vi "SetTextplain.vi"(8 "error in (no error)":errorcluster, 10 "text/plain":string, 11 "object in":refnum<class "execute_result Message.lvclass">) -> (0 "error out":errorcluster, 3 "object out":refnum<class "execute_result Message.lvclass">)   [LabVIEW 2018]
uses:
  execute_result Message.lvclass
  C:/Users/gavin/Documents/LabVIEW Data/LabVIEW-Bits/Connectivity/Jupyter Client/IOPub Messages/display_data Message/display_data Message.lvclass
  C:/Users/gavin/Documents/LabVIEW Data/LabVIEW-Bits/Connectivity/Jupyter Client/Base Classes/Message Class/Message Class.lvclass
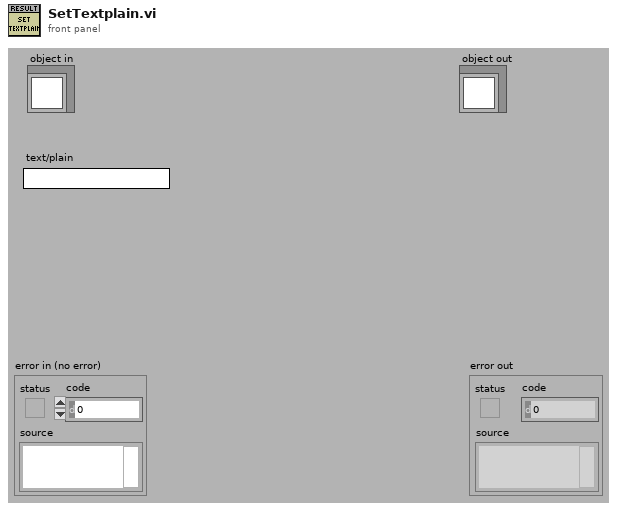
[diagram p1: front panel]
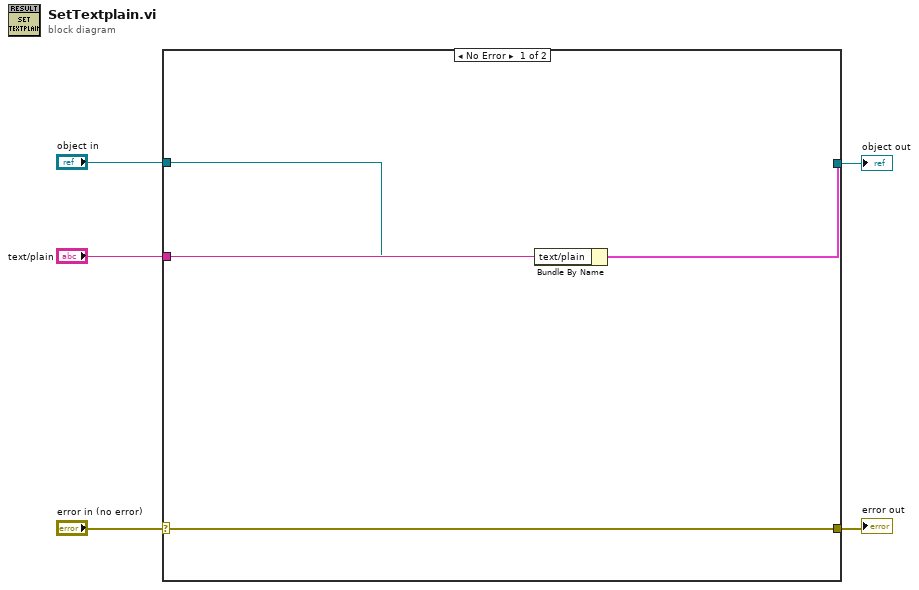
[diagram p0: block diagram]
diagram:
  n1 = case shown="No Error" "error in (no error)" {
    selector: "error in (no error)" -> [w8 w11]
    tunnel: [w8 w11] -> w4
    tunnel: [w6 w10] -> w2
    tunnel: "object in" -> [w7 w10]
    tunnel: "text/plain" -> [w9 _]
    frame No Error {
      n2 = Bundle By Name(cluster=w7, "text/plain"=w9) -> (w6:cluster{})
    }
    frame Error {
    }
  }
  "error out" <- w4
  "object out" <- w2
